vi "Load String Array from File.vi"(7 "Remove empty strings?(T)":bool=TRUE, 11 "File name":string) -> (2 "Success?":bool, 3 "Loaded 1D String Array":string[](array[string]))   [LabVIEW 2019]
uses:
  3df106a3-ef75-4d7e-9d14-752f1648f20a.vi
  <vilib>/Utility/file.llb/Read Delimited Spreadsheet (string).vi
  AutoMenuCreator.lvlib
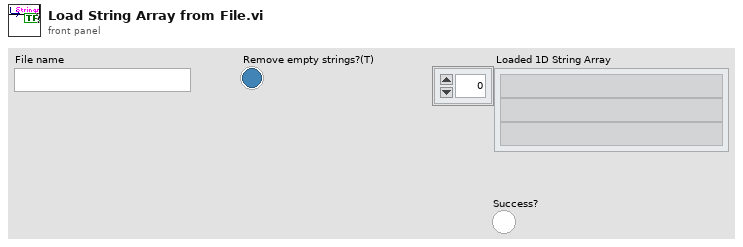
[diagram p1: front panel]
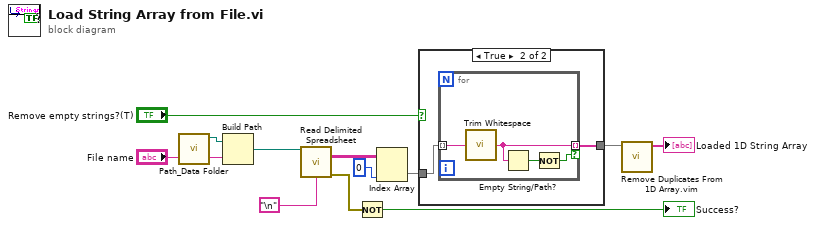
[diagram p0: block diagram]
diagram:
  n1 = call "Path_Data Folder.vi"() -> ("Data Folder Path"=w3:path)  [unwired: 11 in]
  n2 = Build Path(base path=w3, name or relative path="File name") -> (appended path=w6:path)
  n3 = call-poly <vilib>:"Read Delimited Spreadsheet.vi"("file path (dialog if empty)"=w6, "delimiter (\\t)"="\n") -> ("all rows"=w7:string[][], "error out"=w2:errorcluster)  [unwired: 8 in, 4 out]
  n4 = Not(x=w2) -> (.not. x?=→"Success?":bool)
  n5 = Index Array(array=w7, index (col)=0 ("disabled index (col)")) -> (element=w10:string[])  [unwired: 1 in]
  n6 = case shown="True" "Remove empty strings?(T)" {
    tunnel: [w13 w15] -> w11
    tunnel: w10 -> [w13 w14]
    frame False {
    }
    frame True {
      n7 = for {
        tunnel: w14 -> [w19] mode=indexing
        tunnel: [w17] -> w15 mode=indexing if=w16
        n8 = call <vilib>:"Trim Whitespace.vi"("string"=w19) -> ("trimmed string"=w17:string)  [unwired: 1 in]
        n9 = Empty String/Path?(string/path=w17) -> (empty?=w18:bool)
        n10 = Not(x=w18) -> (.not. x?=w16:bool)
      }
    }
  }
  n11 = call "Remove Duplicates From 1D Array.vim"("array"=w11) -> ("array with duplicates removed"=→"Loaded 1D String Array":string[])  [unwired: 10 in]
